vi "ScaleToBuild.vi"(10 "BuildSize":dbl, 11 "Triangles":T1[](array[typedef])) -> (3 "TrianglesOut":T1[](array[typedef]))   [LabVIEW 2014]
uses:
  TypeDefs/TriangleFace.ctl
  TypeDefs/Point3D.ctl
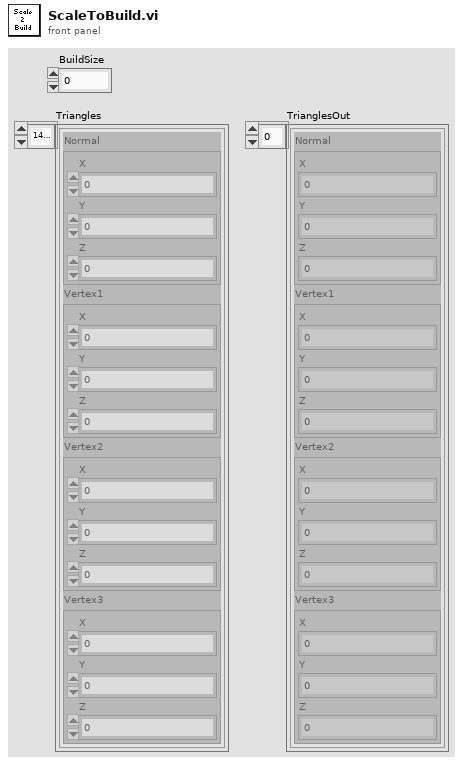
[diagram p1: front panel]
types:
  T1 = typedef "TriangleFace.ctl" = cluster{"Normal":T2, "Vertex1":T2, "Vertex2":T2, "Vertex3":T2}
  T2 = typedef "Point3D.ctl" = cluster{"X":sgl, "Y":sgl, "Z":sgl}
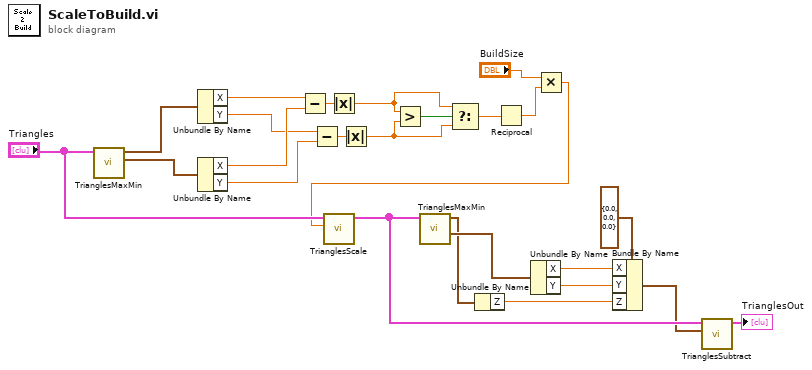
[diagram p0: block diagram]
diagram:
  n1 = call "TrianglesMaxMin.vi"("Triangles"="Triangles") -> ("MaxDims"=w24:T2, "MinDims"=w25:T2)  [unwired: 8 in, 1 out]
  n2 = Unbundle By Name(w25) -> ("X"=w23:sgl, "Y"=w19:sgl)
  n3 = Unbundle By Name(w24) -> ("X"=w22:sgl, "Y"=w18:sgl)
  n4 = Subtract(x=w23, y=w22) -> (x-y=w21:sgl)
  n5 = Subtract(x=w19, y=w18) -> (x-y=w20:sgl)
  n6 = Absolute Value(x=w21) -> (abs(x)=w16:sgl)
  n7 = Absolute Value(x=w20) -> (abs(x)=w15:sgl)
  n8 = Greater?(x=w16, y=w15) -> (0:w17:bool)
  n9 = Select(t=w16, s=w17, f=w15) -> (s? t:f=w13:sgl)
  n10 = Reciprocal(x=w13) -> (1/x=w4:sgl)
  n11 = Multiply(x="BuildSize", y=w4) -> (x*y=w3:dbl)
  n12 = call "TrianglesScale.vi"("ScaleFac"=w3, "TrianglesIn"="Triangles") -> ("TrianglesOut"=w8:T1[])  [unwired: 9 in]
  n13 = call "TrianglesMaxMin.vi"("Triangles"=w8) -> ("Center"=w12:T2, "MinDims"=w2:T2)  [unwired: 8 in, 1 out]
  n14 = Unbundle By Name(w2) -> ("Z"=w1:sgl)
  n15 = Unbundle By Name(w12) -> ("X"=w10:sgl, "Y"=w9:sgl)
  n16 = Bundle By Name(cluster=T2 {"X"=0.0, "Y"=0.0, "Z"=0.0} ("Point3D"), "X"=w10, "Y"=w9, "Z"=w1) -> (w7:T2)
  n17 = call "TrianglesSubtract.vi"("Point3D"=w7, "TrianglesIn"=w8) -> ("TrianglesOut"=→"TrianglesOut":T1[])  [unwired: 9 in]
